vi "Store Configuration Parameters.vi"(8 "error in (no error)":errorcluster, 10 "refnum":T1, 11 "DAQ Configuration in":refnum<class "DAQ Configuration.lvclass">) -> (0 "error out":errorcluster, 2 "refnum out":T1, 3 "DAQ Configuration out":refnum<class "DAQ Configuration.lvclass">)   [LabVIEW 2016, in "Hardware.lvlib" / "DAQ Configuration.lvclass"]
uses:
  DAQ Configuration.lvclass
  <vilib>/Utility/config.llb/Config Data RefNum.ctl
  DAQ Configuration.lvclass/DAQ Configuration.ctl
  HW Config/HW Configuration.lvclass
  <vilib>/Utility/config.llb/NI_LVConfig.lvlib
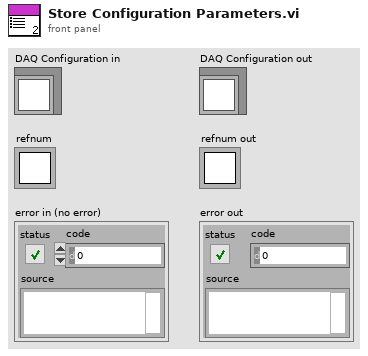
[diagram p1: front panel]
types:
  T1 = typedef "NI_LVConfig.lvlib/Config Data RefNum.ctl" = refnum<k1>
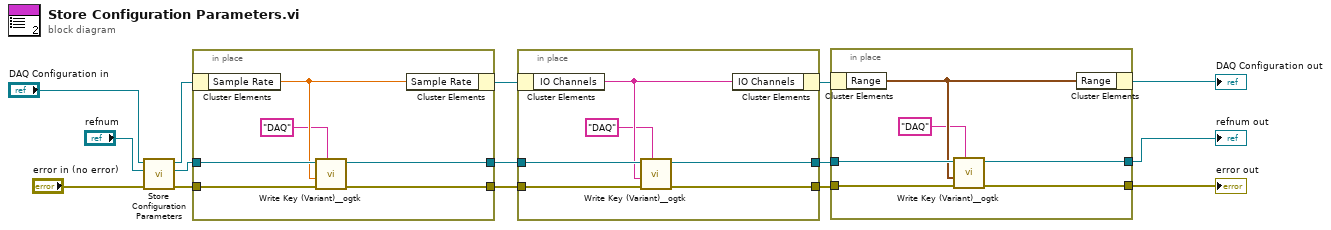
[diagram p0: block diagram]
diagram:
  n1 = call-parent "Store Configuration Parameters.vi"("error in (no error)"="error in (no error)", "refnum"="refnum", "Configuration in"="DAQ Configuration in") -> ("error out"=w10:errorcluster, "refnum out"=w11:T1, "Configuration out"=w12:refnum<class "DAQ Configuration.lvclass">)  [unwired: 6 in]
  n2 = in-place "In Place Element Structure" {
    in-place-border: w11 -> [w21]
    in-place-border: w10 -> [w20]
    in-place-border: [w17] -> w7
    in-place-border: [w16] -> w8
    n3 = in-place-cluster #1(w12) -> ("Sample Rate"=w19:dbl)
    n4 = call <userlib>:"Write Key (Variant)__ogtk.vi"("section"="DAQ", "error in (no error)"=w20, "key-value"=w19, "refnum"=w21) -> ("error out"=w17:errorcluster, "refnum out"=w16:T1)  [unwired: 6 in]
    n5 = in-place-cluster #1("Sample Rate"=w19) -> (w9:refnum<class "DAQ Configuration.lvclass">)
  }
  n6 = in-place "In Place Element Structure" {
    in-place-border: w8 -> [w27]
    in-place-border: w7 -> [w26]
    in-place-border: [w23] -> w5
    in-place-border: [w22] -> w6
    n7 = in-place-cluster #2(w9) -> ("IO Channels"=w25:string)
    n8 = call <userlib>:"Write Key (Variant)__ogtk.vi"("section"="DAQ", "error in (no error)"=w26, "key-value"=w25, "refnum"=w27) -> ("error out"=w23:errorcluster, "refnum out"=w22:T1)  [unwired: 6 in]
    n9 = in-place-cluster #2("IO Channels"=w25) -> (w4:refnum<class "DAQ Configuration.lvclass">)
  }
  n10 = in-place "In Place Element Structure" {
    in-place-border: w6 -> [w33]
    in-place-border: w5 -> [w32]
    in-place-border: [w29] -> w1
    in-place-border: [w28] -> w2
    n11 = in-place-cluster #3(w4) -> ("Range"=w31:cluster{"Ranve (min)":dbl, "Range Max":dbl})
    n12 = call <userlib>:"Write Key (Variant)__ogtk.vi"("section"="DAQ", "error in (no error)"=w32, "key-value"=w31, "refnum"=w33) -> ("error out"=w29:errorcluster, "refnum out"=w28:T1)  [unwired: 6 in]
    n13 = in-place-cluster #3("Range"=w31) -> (→"DAQ Configuration out":refnum<class "DAQ Configuration.lvclass">)
  }
  "error out" <- w1
  "refnum out" <- w2
